vi "Process_input_string.vi"(3 "error in (no error)":errorcluster, 4 "Input":string, 5 "Output_window_old":string) -> (0 "error out":errorcluster, 1 "Result":string, 2 "Output":string)   [LabVIEW 2013]
uses:
  <vilib>/gmath/NI_Gmath.lvlib
panel:
  out "output 2":dbl
  out "Formatted formula string":string
  # "1G*sin(pi)/(pi*22e6*10k*1.25e1)"
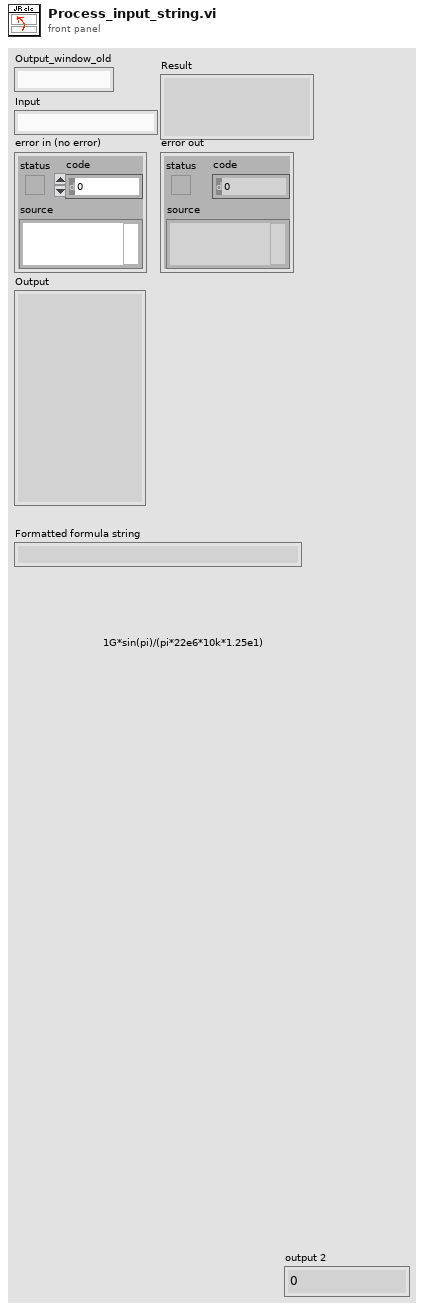
[diagram p1: front panel]
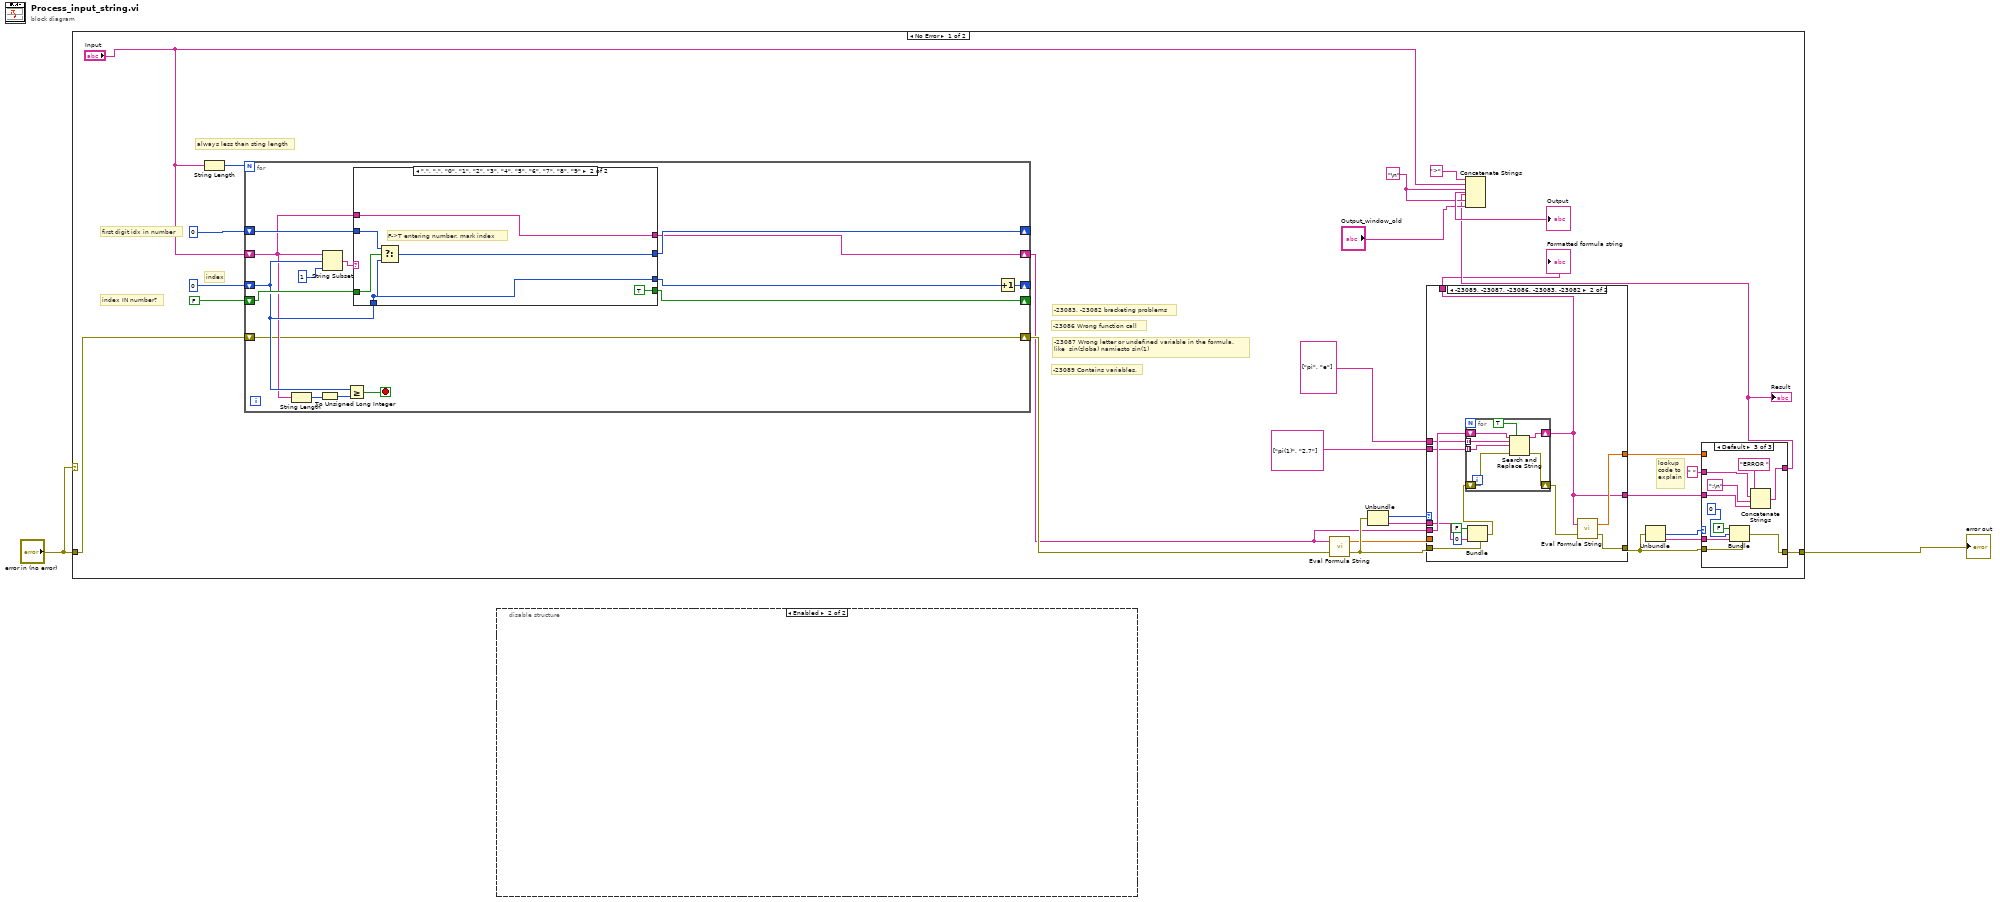
[diagram p0: block diagram]
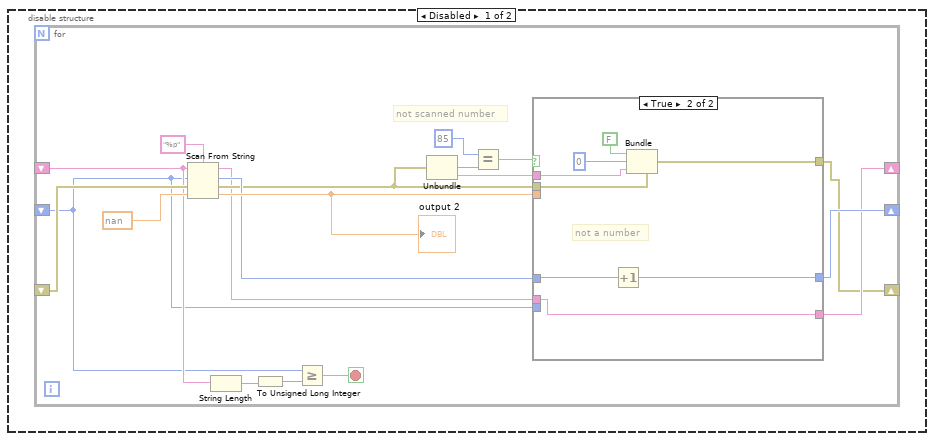
[diagram p2: hidden frame]
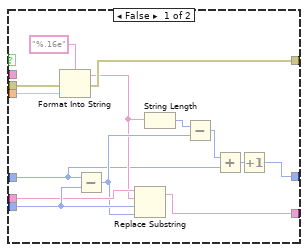
[diagram p3: hidden frame]
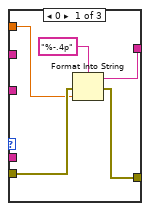
[diagram p4: hidden frame]
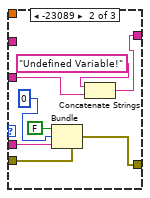
[diagram p5: hidden frame]
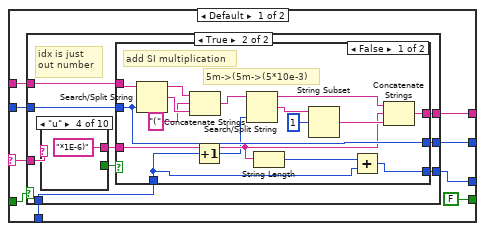
[diagram p7: hidden frame]
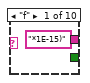
[diagram p9: hidden frame]
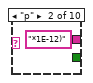
[diagram p10: hidden frame]
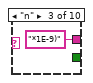
[diagram p11: hidden frame]
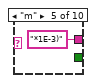
[diagram p12: hidden frame]
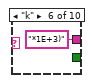
[diagram p13: hidden frame]
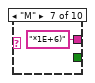
[diagram p14: hidden frame]
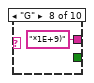
[diagram p15: hidden frame]
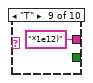
[diagram p16: hidden frame]
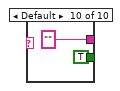
[diagram p17: hidden frame]
diagram:
  n1 = case shown="No Error" "error in (no error)" {
    tunnel: "error in (no error)" -> [w25 w147]
    tunnel: [w12 w147] -> w1
    frame No Error {
      w27 = "\n" ("string")
      # "lookup\ncode to\nexplain"
      # "index IN number?"
      # "first digit idx in number"
      # "index"
      # "-23083, -23082 bracketing problems"
      # "-23086 Wrong function call"
      # "-23089 Contains variables."
      # "-23087 Wrong letter or undefined variable in the formula.\nlike  sin(zloba) namiesto sin(1)"
      # "always less than sting length"
      n2 = String Length(string="Input") -> (length=w23:i32)
      n3 = for {
        N: w23 -> [_]
        shift-right: [w84] -> _
        shift-left: u32 0 ("initial scan location") -> [w81]
        shift-right: [w76] -> w19
        shift-left: "Input" -> [w77]
        shift-right: [w75] -> w21
        shift-left: w25 -> [w75]
        shift-right: [w78] -> _
        shift-left: u32 0 ("initial scan location") -> [w80]
        shift-right: [w82] -> _
        shift-left: FALSE -> [w83]
        stop <- w89 stop-if-true
        n4 = String Length(string=w77) -> (length=w88:i32)
        n5 = To Unsigned Long Integer(number=w88) -> (unsigned 32bit integer=w87:u32)
        n6 = String Subset(string=w77, offset (0)=w81, length (rest)=1 ("length (rest)")) -> (substring=w85:string)
        n7 = Greater Or Equal?(x=w81, y=w87) -> (x >= y?=w89:bool)
        n8 = case shown="\",\", \".\", \"0\", \"1\", \"2\", \"3\", \"4\", \"5\", \"6\", \"7\", \"8\", \"9\"" w85 {
          selector: w85 -> [w96 _]
          tunnel: w83 -> [w97 w145]
          tunnel: [FALSE TRUE] -> w82
          tunnel: w81 -> [w95 w142]
          tunnel: w80 -> [w93 w141]
          tunnel: [w94 w142] -> w79
          tunnel: [w92 w144] -> w78
          tunnel: w77 -> [w91 w143]
          tunnel: [w90 w143] -> w76
          frame Default {
            n9 = case shown="True" w97 {
              tunnel: w96 -> [_ w110]
              tunnel: w95 -> [w100 w108]
              tunnel: [w100 w107] -> w94
              tunnel: w93 -> [w101 w105]
              tunnel: [w101 w104] -> w92
              tunnel: w91 -> [w99 w103]
              tunnel: [w99 w102] -> w90
              frame False {
                # "not in number, not entering or leaving number"
              }
              frame True {
                # "idx is just\nout number"
                n10 = case shown="\"u\"" w110 {
                  tunnel: ["*1E-15)" "*1E-12)" "*1E-9)" "*1E-6)" "*1E-3)" "*1E+3)" "*1E+6)" "*1E+9)" "*1e12)" ""] -> w106
                  tunnel: [_ _ _ _ _ _ _ _ _ TRUE] -> w109
                  frame "f" {
                  }
                  frame "p" {
                  }
                  frame "n" {
                  }
                  frame "u" {
                  }
                  frame "m" {
                  }
                  frame "k" {
                  }
                  frame "M" {
                  }
                  frame "G" {
                  }
                  frame "T" {
                  }
                  frame Default {
                  }
                }
                n11 = case shown="False" w109 {
                  tunnel: w108 -> [w125 w140]
                  tunnel: [w124 w140] -> w107
                  tunnel: w106 -> [w126 _]
                  tunnel: w105 -> [w127 w139]
                  tunnel: [w127 w139] -> w104
                  tunnel: w103 -> [w137 w138]
                  tunnel: [w128 w138] -> w102
                  frame False {
                    # "5m->(5m->(5*10e-3)"
                    # "add SI multiplication"
                    n12 = Search/Split String(string=w137, offset (0)=w127) -> (substring before match=w136:string, match + rest of string=w135:string)  [unwired: 1 in, 1 out]
                    n13 = Concatenate Strings(w136, "(" ("string"), w135) -> (w133:string)
                    n14 = Increment(x=w125) -> (x+1=w122:u32)
                    n15 = Search/Split String(string=w133, offset (0)=w122) -> (substring before match=w132:string, match + rest of string=w131:string)  [unwired: 1 in, 1 out]
                    n16 = String Length(string=w126) -> (length=w123:i32)
                    n17 = String Subset(string=w131, offset (0)=1) -> (substring=w129:string)  [unwired: 1 in]
                    n18 = Add(x=w123, y=w125) -> (x+y=w124:u32)
                    n19 = Concatenate Strings(w132, w126, w129) -> (w128:string)
                  }
                  frame True {
                    # "no SI suffix"
                  }
                }
              }
            }
          }
          frame ",", ".", "0", "1", "2", "3", "4", "5", "6", "7", "8", "9" {
            # "F->T entering number, mark index"
            n20 = Select(t=w141, s=w145, f=w142) -> (s? t:f=w144:u32)
          }
        }
        n21 = Increment(x=w79) -> (x+1=w84:u32)
      }
      n22 = call <vilib>:"Eval Formula String.vi"("error in (no error)"=w21, "formula"=w19) -> ("error out"=w20:errorcluster, "y value"=w15:dbl)
      n23 = Unbundle(w20) -> ("code"=w10:i32, "source"=w18:string)  [unwired: 1 out]
      n24 = case shown="-23089, -23087, -23086, -23083, -23082" w10 {
        tunnel: w20 -> [w55 w64]
        tunnel: [w55 w60] -> w14
        tunnel: w19 -> [w53 w67]
        tunnel: string[] ["pi", "e"] -> [_ w66]
        tunnel: string[] ["pi(1)", "2.7"] -> [_ w65]
        tunnel: w18 -> [_ w63]
        tunnel: [w54 w59] -> w11
        tunnel: w15 -> [w54 _]
        tunnel: [w53 w58] -> w6
        tunnel: [w53 w58] -> w8
        frame 0, Default {
          # "no variables, evaluated correctly"
        }
        frame -23089, -23087, -23086, -23083, -23082 {
          n25 = Bundle(cluster=w64, "status"=FALSE, "code"=0, "source"=w63) -> (w57:errorcluster)
          n26 = for {
            tunnel: w66 -> [w73] mode=indexing
            tunnel: w65 -> [w72] mode=indexing
            shift-right: [w70] -> w58
            shift-left: w67 -> [w74]
            shift-right: [w68] -> w56
            shift-left: w57 -> [w71]
            n27 = Search and Replace String(replace all?=TRUE ("replace all? (F)"), input string=w74, search string=w73, replace string=w72, error in=w71) -> (result string=w70:string, error out=w68:errorcluster)  [unwired: 3 in, 2 out]
          }
          n28 = call <vilib>:"Eval Formula String.vi"("error in (no error)"=w56, "formula"=w58) -> ("error out"=w60:errorcluster, "y value"=w59:dbl)
        }
      }
      "Formatted formula string" <- w6
      n29 = Unbundle(w14) -> ("code"=w9:i32, "source"=w13:string)  [unwired: 1 out]
      n30 = case shown="Default" w9 {
        tunnel: w14 -> [w32 w39 w50]
        tunnel: w13 -> [_ w40 w45]
        tunnel: [w33 w36 w47] -> w7
        tunnel: [w31 w38 w49] -> w12
        tunnel: w11 -> [w30 _ _]
        tunnel: w8 -> [_ w35 w46]
        tunnel: " " ("format string") -> [_ _ w43]
        frame 0 {
          n31 = Format Into String(format string="%-.4p", error in=w32, w30) -> (resulting string=w33:string, error out=w31:errorcluster)  [unwired: 1 in]
        }
        frame -23089 {
          n32 = Bundle(cluster=w39, "status"=FALSE, "code"=0, "source"=w40) -> (w38:errorcluster)
          n33 = Concatenate Strings("Undefined Variable!" ("format string"), w35) -> (w36:string)
        }
        frame Default {
          n34 = Bundle(cluster=w50, "status"=FALSE, "code"=0, "source"=w45) -> (w49:errorcluster)
          n35 = Concatenate Strings("ERROR " ("format string"), w43, ":\n" ("format string"), w46) -> (w47:string)
        }
      }
      "Result" <- w7
      n36 = Concatenate Strings(">" ("string"), "Input", w27, w7, w27, "Output_window_old") -> (→"Output":string)
    }
    frame Error {
    }
  }
  "error out" <- w1
  n37 = disable-structure shown="Enabled" {
    frame Disabled {
      n38 = for {
        shift-right: [w156] -> _
        shift-left: _ -> [w149]
        shift-right: [w155] -> _
        shift-left: _ -> [w153]
        shift-right: [w148] -> _
        shift-left: _ -> [w163]
        stop <- w152 stop-if-true
        # "not scanned number"
        n39 = Scan From String(format string="%p", input string=w153, initial scan location=w149, error in=w163, default 1=nan ("default value 1")) -> (offset past scan=w162:u32, error out=w154:errorcluster, output 1=w164:dbl)  [unwired: 1 out]
        "output 2" <- w164
        n40 = String Length(string=w153) -> (length=w151:i32)
        n41 = To Unsigned Long Integer(number=w151) -> (unsigned 32bit integer=w150:u32)
        n42 = Greater Or Equal?(x=w149, y=w150) -> (x >= y?=w152:bool)
        n43 = Unbundle(w154) -> ("code"=w158:i32, "source"=w157:string)  [unwired: 1 out]
        n44 = Equal?(x=85, y=w158) -> (x = y?=w159:bool)
        n45 = case shown="True" w159 {
          tunnel: w164 -> [w179 _]
          tunnel: w162 -> [w167 w182]
          tunnel: w149 -> [w178 _]
          tunnel: w153 -> [w177 w183]
          tunnel: [w176 w183] -> w155
          tunnel: w154 -> [w175 w187]
          tunnel: w157 -> [_ w185]
          tunnel: [w173 w184] -> w148
          tunnel: [w166 w181] -> w156
          frame False {
            n46 = Format Into String(format string="%.16e", error in=w175, w179) -> (resulting string=w170:string, error out=w173:errorcluster)  [unwired: 1 in]
            n47 = Subtract(x=w167, y=w178) -> (x-y=w172:u32)
            n48 = Replace Substring(2:w172, 3:w178, 4:w170, 5:w177) -> (1:w176:string)  [unwired: 1 out]
            n49 = String Length(string=w170) -> (length=w171:i32)
            n50 = Subtract(x=w171, y=w172) -> (x-y=w168:u32)
            n51 = Add(x=w168, y=w167) -> (x+y=w169:u32)
            n52 = Increment(x=w169) -> (x+1=w166:u32)
          }
          frame True {
            # "not a number"
            n53 = Increment(x=w182) -> (x+1=w181:u32)
            n54 = Bundle(cluster=w187, "status"=FALSE, "code"=0, "source"=w185) -> (w184:errorcluster)
          }
        }
      }
    }
    frame Enabled {
    }
  }
